vi "Local Configuration.Get Register Offset.vi"(11 "Local Configuration Register":T1) -> (3 "Offset":u32)   [LabVIEW 2016, in "GE 5565PIORC.lvclass"]
uses:
  GE 5565PIORC.lvclass
  Controls/Registers.Local Configuration.ctl
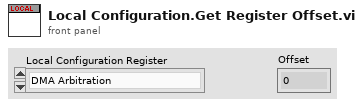
[diagram p1: front panel]
types:
  T1 = typedef "GE 5565PIORC.lvclass/Registers.Local Configuration.ctl" = enum16{"DMA Arbitration", "Interrupt Control and Status", "DMA Mode", "DMA PCI Address", "DMA Local Address", "DMA Transfer Size", "DMA Descriptor Pointer", "DMA Command/Status", "DMA PCI DAC Upper Address", "PCI PIO Address Range", "PCI PIO Base Address (Remap)"}
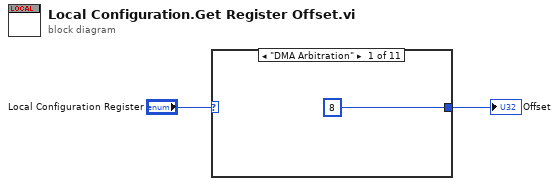
[diagram p0: block diagram]
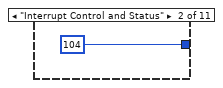
[diagram p2: hidden frame]
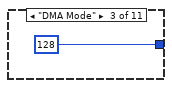
[diagram p3: hidden frame]
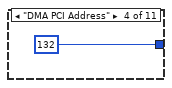
[diagram p4: hidden frame]
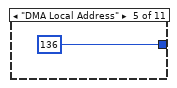
[diagram p5: hidden frame]
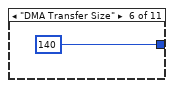
[diagram p6: hidden frame]
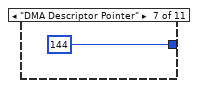
[diagram p7: hidden frame]
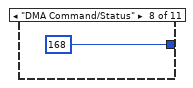
[diagram p8: hidden frame]
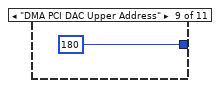
[diagram p9: hidden frame]
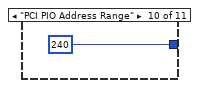
[diagram p10: hidden frame]
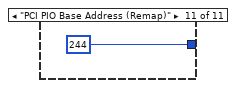
[diagram p11: hidden frame]
diagram:
  n1 = case shown="\"DMA Arbitration\"" "Local Configuration Register" {
    tunnel: [u32 8 u32 104 u32 128 u32 132 u32 136 u32 140 u32 144 u32 168 u32 180 u32 240 u32 244] -> w1
    frame "DMA Arbitration" {
    }
    frame "Interrupt Control and Status" {
    }
    frame "DMA Mode" {
    }
    frame "DMA PCI Address" {
    }
    frame "DMA Local Address" {
    }
    frame "DMA Transfer Size" {
    }
    frame "DMA Descriptor Pointer" {
    }
    frame "DMA Command/Status" {
    }
    frame "DMA PCI DAC Upper Address" {
    }
    frame "PCI PIO Address Range" {
    }
    frame "PCI PIO Base Address (Remap)" {
    }
  }
  "Offset" <- w1
